vi "init_task.vi"(6 "number of samples":i32=1000, 7 "rate":dbl=5000.0, 8 "error in":errorcluster, 10 "input terminal configuration":i32(ring)=10106 items=["default"=-1, "RSE"=10083, "NRSE"=10078, "Differential"=10106, "Pseudodifferential"=12529], 11 "device channel list":string[](array[string])) -> (0 "error out":errorcluster, 3 "task out":refnum<k21>)   [LabVIEW 2016]
uses:
  <vilib>/DAQmx/configure/timing.llb/DAQmx Timing (Sample Clock).vi
  <vilib>/DAQmx/create/channels.llb/DAQmx Create Channel (AI-Voltage-Basic).vi
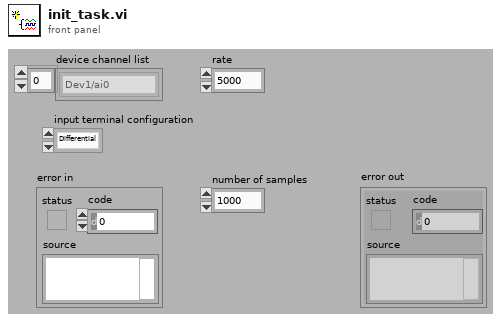
[diagram p1: front panel]
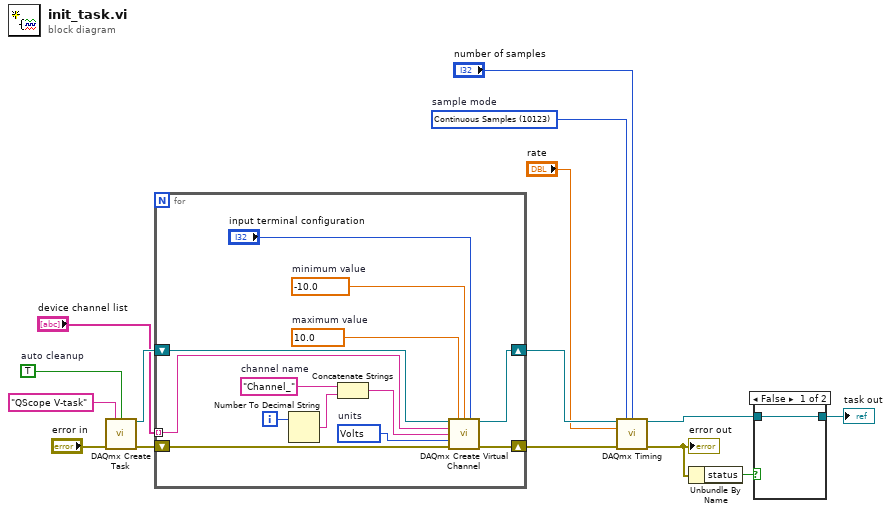
[diagram p0: block diagram]
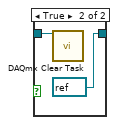
[diagram p2: hidden frame]
diagram:
  w11 = 10123 items=["Finite Samples"=10178, "Continuous Samples"=10123, "Hardware Timed Single Point"=12522]  # sample mode
  w13 = TRUE  # auto cleanup
  n1 = call <vilib>:"DAQmx Create Task.vi"("new task name"="QScope V-task", "auto cleanup"=w13, "error in"="error in") -> ("task out"=w12:refnum<k21>, "error out"=w14:errorcluster)  [unwired: 11 in]
  n2 = for {
    shift-right: [w24] -> w7
    shift-left: w14 -> [w28]
    shift-right: [w22] -> w8
    shift-left: w12 -> [w27]
    tunnel: "device channel list" -> [w21] mode=indexing
    i -> [w20]
    w23 = 10348 items=["Volts"=10348, "From Custom Scale"=10065]  # units
    w18 = "Channel_"  # channel name
    w25 = -10.0  # minimum value
    w26 = 10.0  # maximum value
    n3 = Number To Decimal String(number=w20) -> (decimal integer string=w19:string)  [unwired: 1 in]
    n4 = Concatenate Strings(w18, w19) -> (w17:string)
    n5 = call-poly <vilib>:"DAQmx Create Virtual Channel.vi"("task in"=w27, "maximum value"=w26, "minimum value"=w25, "input terminal configuration"="input terminal configuration", "physical channels"=w21, "name to assign"=w17, "units"=w23, "error in"=w28) -> ("task out"=w22:refnum<k21>, "error out"=w24:errorcluster)  [unwired: 6 in]
  }
  n6 = call-poly <vilib>:"DAQmx Timing.vi"("task/channels in"=w8, "sample mode"=w11, "samples per channel"="number of samples", "rate"="rate", "error in"=w7) -> ("task out"=w2:refnum<k21>, "error out"=w4:errorcluster)  [unwired: 9 in]
  "error out" <- w4
  n7 = Unbundle By Name(w4) -> ("status"=w3:bool)
  n8 = case shown="False" w3 {
    tunnel: w2 -> [w29 w31]
    tunnel: [w29 refnum<k21> refnum ("task out")] -> w1
    frame False {
    }
    frame True {
      n9 = call <vilib>:"DAQmx Clear Task.vi"("task in"=w31) -> ()  [unwired: 14 in, 1 out]
    }
  }
  "task out" <- w1
